vi "Roller Motor Logic.vi"(6 "Reset?":bool, 11 "Command in":enum16{"Stop", "Forward", "Reverse"}(ring)) -> (1 "Solenoid out":bool, 3 "Command out":enum16{"Stop", "Forward", "Reverse"}(ring))   [LabVIEW 2013]
uses:
  Common Code/Change Detect Boolean.vi
  Robot Global Data.vi
panel:
  in  "Roller sustain time":dbl
  # "Debug controls under this box"
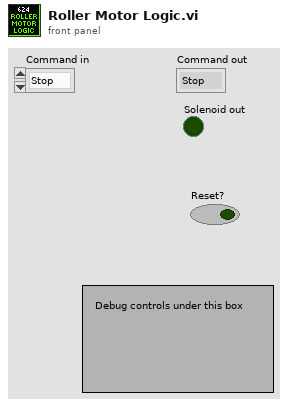
[diagram p1: front panel]
types:
  T1 = typedef "Dashboard UDP Packet.ctl" = cluster{"Camera":T2, "Gyro":T3, "Encoder":T4, "Auto Shift":T5, "Auton":T6, "Drive/Ramp X":dbl, "Drive/Ramp Y":dbl, "Drive/Battery Cutoff":dbl, "Pressure/Compressor Min Voltage":dbl, "Pressure/Compressor Delay":dbl, "Controller/Strafe Correction":bool, "Shooter":T7, "Rollers":T8, "Abort":bool, "Finish":bool}
  T2 = typedef "Camera Controls.ctl" = cluster{"Camera/View Angle X":dbl, "Camera/Goal Track Timeout":dbl, "Camera/View Angle Y":dbl, "Camera/Goal Exposure":dbl, "Camera/Vision Receive Timeout":dbl, "Camera/Offset 1":dbl, "Camera/Offset 2":dbl}
  T3 = typedef "Gyro Controls.ctl" = cluster{"Gyro/Steer Close PID P":dbl, "Gyro/Steer Close PID I":dbl, "Gyro/Steer Close PID D":dbl, "Gyro/Steer Close PID min":dbl, "Gyro/Steer Close PID max":dbl, "Gyro/Steer PID P":dbl, "Gyro/Steer PID I":dbl, "Gyro/Steer PID D":dbl, "Gyro/Steer PID min":dbl, "Gyro/Angle Tolerance":dbl, "Gyro/Steer PID max":dbl, "Gyro/Steer Closeness Threshold":dbl}
  T4 = typedef "Encoder Controls.ctl" = cluster{"Encoders/Reset":bool, "Encoders/Omni Constant":dbl, "Encoders/Omni Tick Constant":dbl, "Encoders/Left Constant":dbl, "Encoders/Right Constant":dbl, "Encoders/Right Tick Constant":dbl}
  T5 = typedef "Auto Shift Controls.ctl" = cluster{"AutoShift/Upshift Throttle Accel":dbl, "AutoShift/Speed Threshold":dbl, "AutoShift/Upshift Throttle":dbl, "AutoShift/Upshift Accel":dbl, "AutoShift/Downshift Accel":dbl, "AutoShift/Downshift Throttle":dbl, "AutoShift/Delay":dbl, "AutoShift/Enabled":bool}
  T6 = typedef "Auton Controls.ctl" = cluster{"Auton/Left Shoot X-Coord":dbl, "Auton/Right Shoot X-Coord":dbl, "DistDrive/Distance Stop Threshold":dbl, "DistDrive/Max Stop Speed":dbl, "Auton/Back Piston Time":dbl, "Auton/Manual Hot":bool, "Auton/Manual Hot Right":bool, "Auton/X Distance PID max":dbl, "Auton/X Distance PID min":dbl, "Auton/X Distance PID P":dbl, "Auton/X Distance PID I":dbl, "Auton/X Distance PID D":dbl, "Auton/Y Distance PID max":dbl, "Auton/Y Distance PID min":dbl, "Auton/Y Distance PID P":dbl, "Auton/Y Distance PID I":dbl, "Auton/Y Distance PID D":dbl}
  T7 = typedef "Shooter Controls.ctl" = cluster{"Shooter/Reset Time":dbl, "Shooter/Release Delay":dbl, "Shooter/Pressure Steady Time":dbl, "Shooter/Misfire Delay":dbl, "Shooter/Ball Settle Time":dbl, "Shooter/Line IR Delay":dbl, "Pressure/Upper PSI Time":dbl, "Pressure/Lower PSI Time":dbl, "Shooter/Punch Delay":dbl, "Shooter/Target Pressure":dbl, "Pressure/Line B":dbl, "Pressure/Line M":dbl, "Pressure/Shooter M":dbl, "Pressure/Shooter B":dbl}
  T8 = typedef "Roller Controls.ctl" = cluster{"Roller/Load IRs Verify Time":dbl, "Roller/Center IR Latch Time":dbl, "Roller/Speed Front":dbl, "Roller/Speed Back":dbl, "Roller/Entry Timeout":dbl, "Roller/To Center Timeout":dbl, "Roller/Sustain Time":dbl, "Roller/Verify Center Time":dbl}
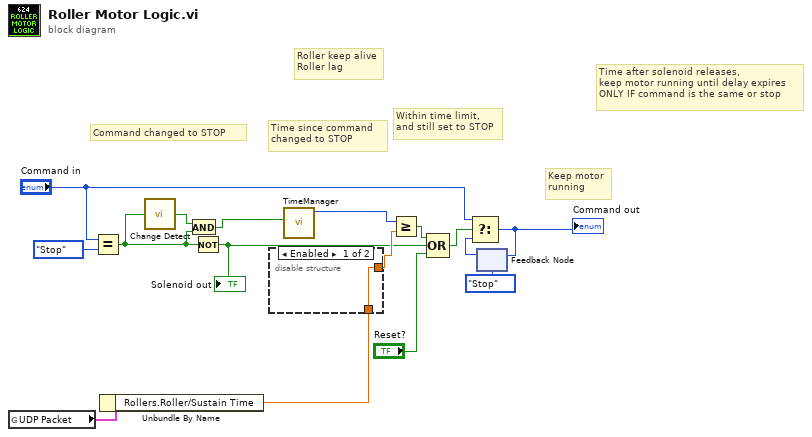
[diagram p0: block diagram]
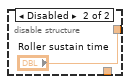
[diagram p2: hidden frame]
diagram:
  # "Keep motor\nrunning"
  # "Within time limit,\nand still set to STOP"
  # "Time since command\nchanged to STOP"
  # "Command changed to STOP"
  # "Time after solenoid releases,\nkeep motor running until delay expires\nONLY IF command is the same or stop"
  # "Roller keep alive\nRoller lag"
  n1 = global read "Robot Global Data.vi" "UDP Packet"() -> (w2:T1)
  n2 = Equal?(x="Command in", y=enum16{"Stop", "Forward", "Reverse"}."Stop") -> (x = y?=w8:bool)
  n3 = Unbundle By Name(w2) -> ("Rollers.Roller/Sustain Time"=w1:dbl)
  n4 = call-poly "Change Detect.vi"("In"=w8) -> ("Changed?"=w15:bool)
  n5 = And(x=w15, y=w8) -> (x .and. y?=w6:bool)
  n6 = Not(x=w8) -> (.not. x?=w4:bool)
  "Solenoid out" <- w4
  n7 = disable-structure shown="Enabled" {
    disable-tunnel: [w17 "Roller sustain time"] -> w7
    disable-tunnel: w1 -> [w17 _]
    frame Enabled {
    }
    frame Disabled {
    }
  }
  n8 = call "TimeManager.vi"("Reset?"=w6) -> ("Time Since Reset"=w5:u32)  [unwired: 9 in, 1 out]
  n9 = Greater Or Equal?(x=w5, y=w7) -> (x >= y?=w10:bool)
  n10 = Compound Arithmetic op=OR(w10, w4, "Reset?") -> (w9:bool)
  n11 = feedback #1(enum16{"Stop", "Forward", "Reverse"}."Stop" ("y")) -> (w13:enum16{"Stop", "Forward", "Reverse"})
  n12 = Select(t="Command in", s=w9, f=w13) -> (s? t:f=w12:enum16{"Stop", "Forward", "Reverse"})
  "Command out" <- w12
  n13 = feedback-in #1(w12) -> ()
